vi "Error Dialog.vi"(6 "Modal (T)":bool=TRUE, 8 "error in (no error)":errorcluster, 10 "Dialog Type":T1) -> (0 "error out":errorcluster)   [LabVIEW 2017, in "Error Dialog w Copy to Clipboard.lvlib"]
doc: "Displays error message to the user.\n\nCopyright (c) 2022, Neosoft Technologies Inc\nAll rights reserved."
uses:
  Error Dialog w Copy to Clipboard.lvlib
  Dialog Type.ctl
  <vilib>/Utility/error.llb/DialogType.ctl
  <vilib>/Platform/browser.llb/Open URL in Default Browser (string).vi
panel:
  out "String":string
  in  "Stop":bool
  in  "Continue":bool
  out "Error Code":string
  in  "Show details":bool
  in  "Screenshot":bool
  in  "URL":bool
  in  "Copy":bool
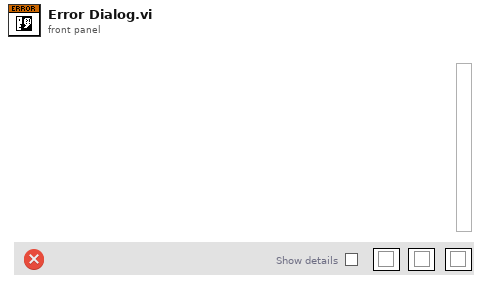
[diagram p1: front panel]
types:
  T1 = typedef "Error Dialog w Copy to Clipboard.lvlib/Dialog Type.ctl" = enum16{"OK message", "Continue or Stop message"}
  T2 = enum32{"Invalid", "Default", "Floating", "Floating/Auto-Hide", "Modal"}
  T3 = enum32{"Invalid", "Standard", "Closed", "Hidden", "Minimized", "Maximized"}
  T4 = cluster{"call chain":string[], "error":errorcluster, "show details":bool, "message":string, "stop":bool}
  T5 = typedef "imagedata.ctl" = cluster{"image type":i32, "image depth":i32, "image":u8[], "mask":u8[], "colors":u32[], "Rectangle":cluster{"left":i16, "top":i16, "right":i16, "bottom":i16}}
  T6 = typedef "DialogType.ctl" = u16
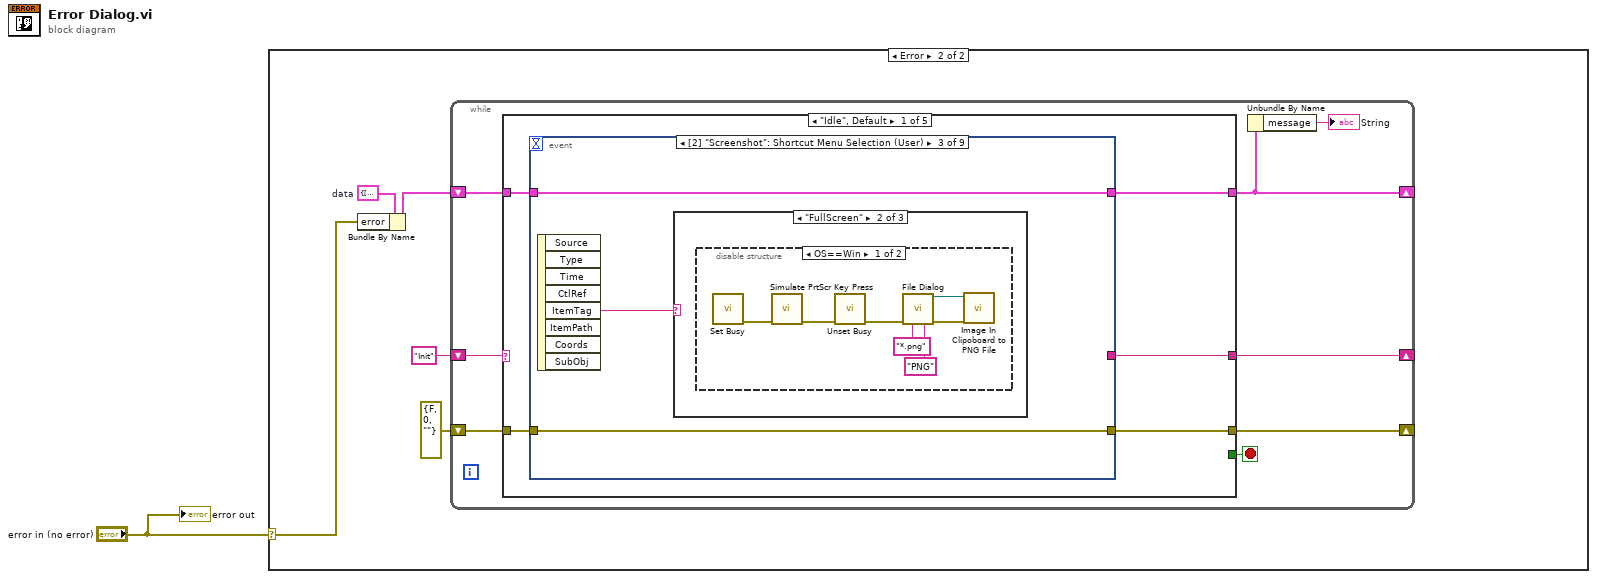
[diagram p0: block diagram]
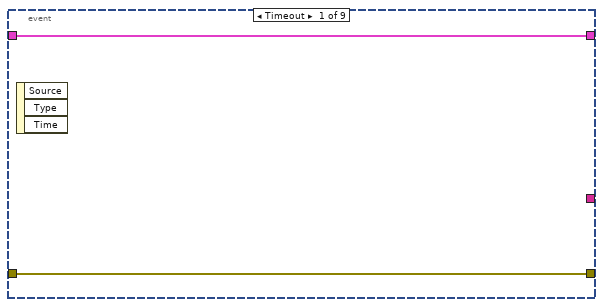
[diagram p3: hidden frame]
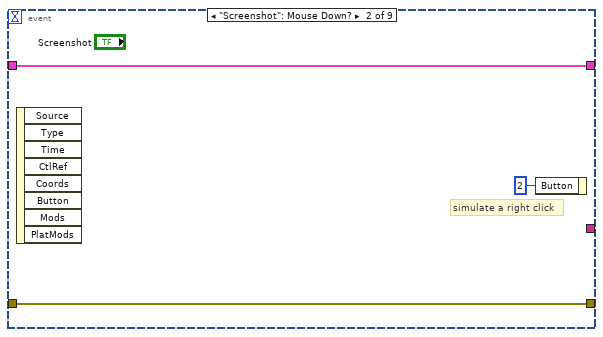
[diagram p4: hidden frame]
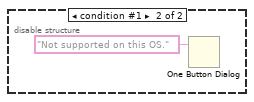
[diagram p6: hidden frame]
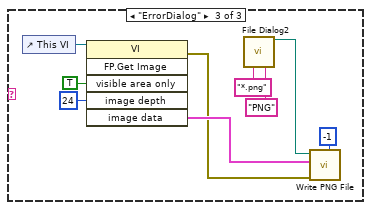
[diagram p7: hidden frame]
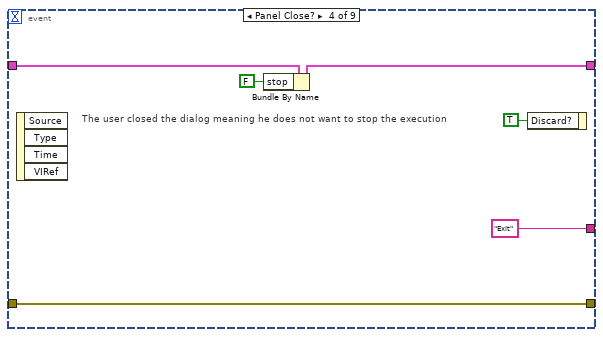
[diagram p8: hidden frame]
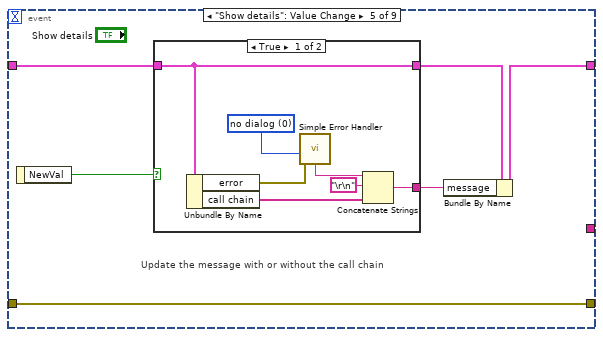
[diagram p9: hidden frame]
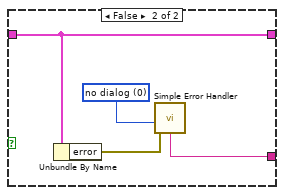
[diagram p10: hidden frame]
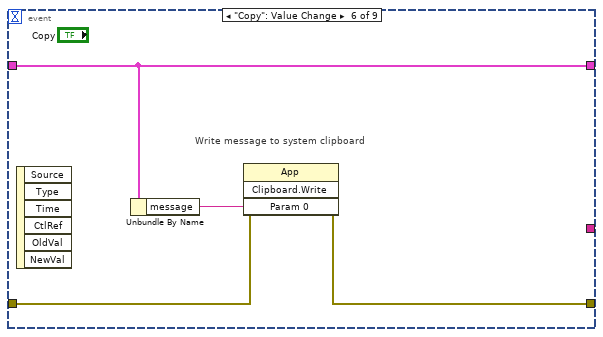
[diagram p11: hidden frame]
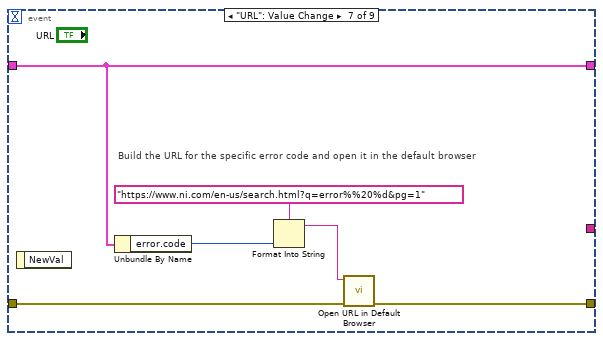
[diagram p12: hidden frame]
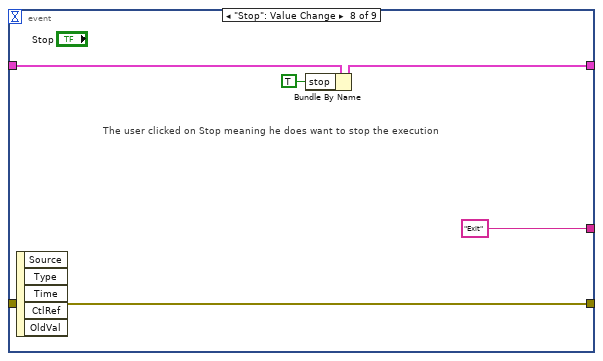
[diagram p13: hidden frame]
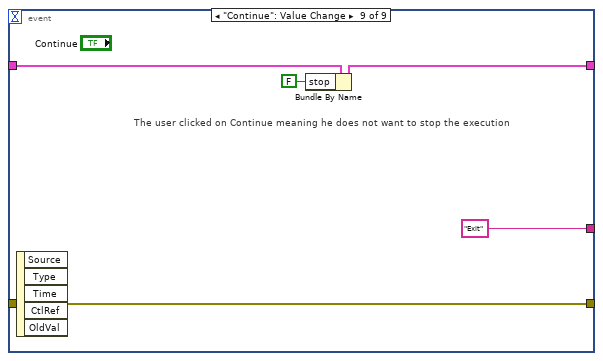
[diagram p14: hidden frame]
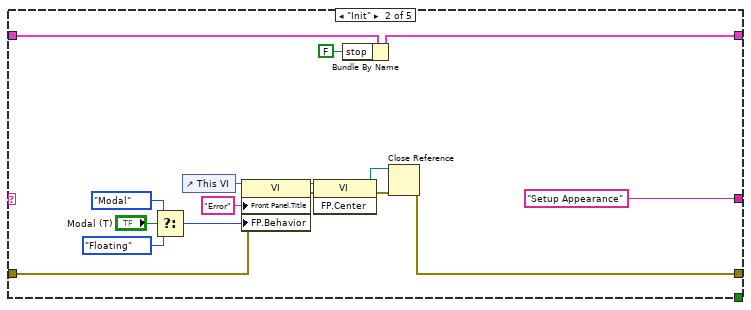
[diagram p15: hidden frame]
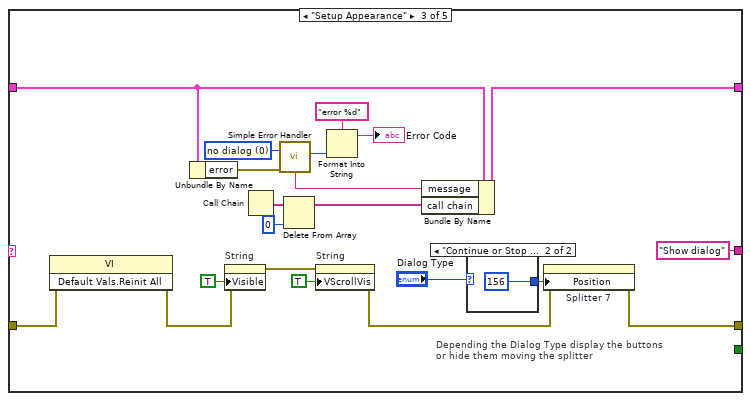
[diagram p16: hidden frame]
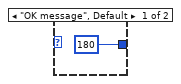
[diagram p17: hidden frame]
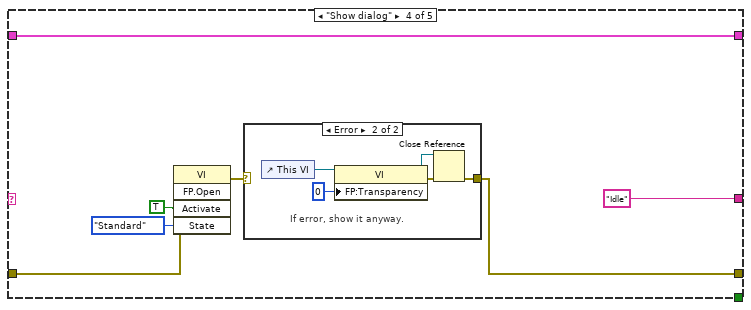
[diagram p18: hidden frame]
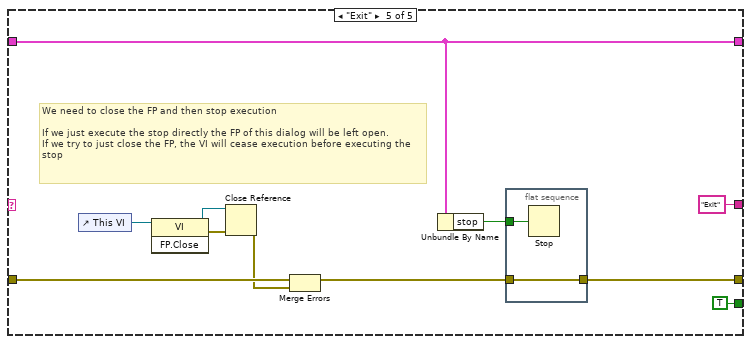
[diagram p20: hidden frame]
diagram:
  n1 = case shown="Error" "error in (no error)" {
    selector: "error in (no error)" -> [_ w3]
    frame No Error {
    }
    frame Error {
      w5 = T4 {"call chain"=[], "error"={"status"=FALSE, "code"=0, "source"=""}, "show details"=FALSE, "message"="", "stop"=FALSE}  # data
      n2 = Bundle By Name(cluster=w5, "error"=w3) -> (w4:T4)
      n3 = while {
        shift-right: [w12] -> _
        shift-left: "Init" ("format string") -> [w13]
        shift-right: [w11] -> _
        shift-left: errorcluster {"status"=FALSE, "code"=0, "source"=""} ("error out") -> [w10]
        shift-right: [w8] -> _
        shift-left: w4 -> [w9]
        stop <- w14 stop-if-true
        n4 = case shown="\"Idle\", Default" w13 {
          tunnel: [_ _ _ _ TRUE ("Discard?")] -> w14
          tunnel: [w15 "Setup Appearance" "Show dialog" "Idle" "Exit" ("format string")] -> w12
          tunnel: [w18 w96 w104 w127 w142] -> w11
          tunnel: w10 -> [w19 w95 w109 w128 w149]
          tunnel: [w16 w89 w115 w133 w144] -> w8
          tunnel: w9 -> [w17 w94 w123 w133 w144]
          frame "Idle", Default {
            n5 = event shown="[2] \"Screenshot\": Shortcut Menu Selection (User)" {
              selector: _ -> [_ _ _ _ _ _ _ _ _]
              dyn-events: _ -> [_ _ _ _ _ _ _ _ _]
              timeout: _ -> [_ _ _ _ _ _ _ _ _]
              tunnel: w19 -> [w21 w22 w27 w50 w56 w69 w73 w82 w87]
              tunnel: [w21 w22 w27 w50 w56 w68 w72 w82 w87] -> w18
              tunnel: w17 -> [w20 w24 w26 w49 w54 w71 w77 w81 w86]
              tunnel: [w20 w24 w26 w46 w52 w71 w77 w80 w85] -> w16
              tunnel: [_ _ _ "Exit" ("format string") _ _ _ "Exit" ("format string") "Exit" ("format string")] -> w15
              event Timeout {
                n6 = event-data() -> ()  [unwired: 1 in, 3 out]
              }
              event "Screenshot": Mouse Down? {
                # "simulate a right click"
                n7 = event-data() -> ()  [unwired: 1 in, 8 out]
                n8 = event-data("Button"=u16 2) -> ()  [unwired: 1 in, 1 out]
              }
              event "Screenshot": Shortcut Menu Selection (User) {
                n9 = event-data() -> ("ItemTag"=w25:string)  [unwired: 1 in, 7 out]
                n10 = case shown="\"FullScreen\"" w25 {
                  frame "False", Default {
                  }
                  frame "FullScreen" {
                    n11 = disable-structure shown="OS==Win" {
                      frame condition #0 (active) {
                        n12 = call <vilib>:"Set Busy.vi"() -> ("error out"=w30:errorcluster)  [unwired: 10 in, 1 out]
                        n13 = call "Simulate PrtScr Key Press.vi"("error in (no error)"=w30) -> ("error out"=w29:errorcluster)  [unwired: 10 in]
                        n14 = call <vilib>:"Unset Busy.vi"("error in (no error)"=w29) -> ("error out"=w28:errorcluster)  [unwired: 10 in]
                        n15 = call "File Dialog"("error in"=w28, "pattern (all files)"="*.png", "pattern label"="PNG") -> ("selected path"=w34:path, "error out"=w31:errorcluster)  [unwired: 9 in, 2 out]
                        n16 = call "Image In Clipoboard to PNG File.vi"("error in (no error)"=w31, "Image Path"=w34) -> ()  [unwired: 9 in, 1 out]
                      }
                      frame condition #1 {
                        n17 = One Button Dialog(message="Not supported on this OS.") -> ()  [unwired: 1 in, 1 out]
                      }
                    }
                  }
                  frame "ErrorDialog" {
                    n18 = control-ref of="This VI"() -> (w44:refnum<vi>)
                    n19 = invoke class="VI" method="FP.Get Image"(reference=w44, "visible area only"=TRUE ("Visible Area Only"), "image depth"=24 ("Image Depth")) -> (error out=w42:errorcluster, "image data"=w43:T5)  [unwired: 3 in, 4 out]
                    n20 = call "File Dialog2"("pattern (all files)"="*.png", "pattern label"="PNG") -> ("selected path"=w36:path)  [unwired: 10 in, 3 out]
                    n21 = call <vilib>:"Write PNG File.vi"("compression (default)"=-1, "error in (no error)"=w42, "image data"=w43, "path to PNG file"=w36) -> ()  [unwired: 6 in, 2 out]
                  }
                }
              }
              event Panel Close? {
                # "The user closed the dialog meaning he does not want to stop the execution"
                n22 = event-data() -> ()  [unwired: 1 in, 4 out]
                n23 = Bundle By Name(cluster=w49, "stop"=FALSE) -> (w46:T4)
                n24 = event-data("Discard?"=TRUE) -> ()  [unwired: 1 in, 1 out]
              }
              event "Show details": Value Change {
                # "Update the message with or without the call chain"
                n25 = event-data() -> ("NewVal"=w55:bool)  [unwired: 1 in]
                n26 = case shown="True" w55 {
                  tunnel: w54 -> [w61 w65]
                  tunnel: [w61 w65] -> w53
                  tunnel: [w57 w64] -> w51
                  frame True {
                    w60 = "\r\n"
                    w63 = T6 0 items=["no dialog", "OK message", "continue or stop message", "OK message + warnings", "continue/stop + warnings"] ("type of dialog (OK msg:1)")
                    n27 = Unbundle By Name(w61) -> ("error"=w62:errorcluster, "call chain"=w58:string[])
                    n28 = call <vilib>:"Simple Error Handler.vi"("type of dialog (OK msg:1)"=w63, "error in (no error)"=w62) -> ("message"=w59:string)  [unwired: 3 in, 4 out]
                    n29 = Concatenate Strings(w59, w60, w60, w58) -> (w57:string)
                  }
                  frame False {
                    w67 = T6 0 items=["no dialog", "OK message", "continue or stop message", "OK message + warnings", "continue/stop + warnings"] ("type of dialog (OK msg:1)")
                    n30 = Unbundle By Name(w65) -> ("error"=w66:errorcluster)
                    n31 = call <vilib>:"Simple Error Handler.vi"("type of dialog (OK msg:1)"=w67, "error in (no error)"=w66) -> ("message"=w64:string)  [unwired: 3 in, 4 out]
                  }
                }
                n32 = Bundle By Name(cluster=w53, "message"=w51) -> (w52:T4)
              }
              event "Copy": Value Change {
                # "Write message to system clipboard"
                n33 = event-data() -> ()  [unwired: 1 in, 6 out]
                n34 = Unbundle By Name(w71) -> ("message"=w70:string)
                n35 = invoke class="App" method="Clipboard.Write"(error in=w69, "Param 0"=w70) -> (error out=w68:errorcluster)  [unwired: 2 in, 3 out]
              }
              event "URL": Value Change {
                # "Build the URL for the specific error code and open it in the default browser"
                n36 = event-data() -> ()  [unwired: 1 in, 1 out]
                n37 = Unbundle By Name(w77) -> ("error.code"=w75:i32)
                n38 = Format Into String(format string="https://www.ni.com/en-us/search.html?q=error%%20%d&pg=1", w75) -> (resulting string=w74:string)  [unwired: 2 in, 1 out]
                n39 = call-poly <vilib>:"Open URL in Default Browser.vi"("error in (no error)"=w73, "URL"=w74) -> ("error out"=w72:errorcluster)  [unwired: 4 in, 1 out]
              }
              event "Stop": Value Change {
                # "The user clicked on Stop meaning he does want to stop the execution"
                n40 = event-data() -> ()  [unwired: 1 in, 5 out]
                n41 = Bundle By Name(cluster=w81, "stop"=TRUE) -> (w80:T4)
              }
              event "Continue": Value Change {
                # "The user clicked on Continue meaning he does not want to stop the execution"
                n42 = event-data() -> ()  [unwired: 1 in, 5 out]
                n43 = Bundle By Name(cluster=w86, "stop"=FALSE) -> (w85:T4)
              }
            }
          }
          frame "Init" {
            n44 = Select(t=T2."Modal" ("Front Panel Window:Behavior"), s="Modal (T)", f=T2."Floating") -> (s? t:f=w90:T2)
            n45 = control-ref of="This VI"() -> (w101:refnum<vi>)
            n46 = property class="VI"(reference=w101, error in=w95, "Front Panel.Title"="Error" ("Front Panel Window:Title"), "FP.Behavior"=w90) -> (reference out=w102:refnum<vi>, error out=w103:errorcluster)
            n47 = invoke class="VI" method="FP.Center"(reference=w102, error in=w103) -> (reference out=w99:refnum<vi>, error out=w98:errorcluster)  [unwired: 1 in, 1 out]
            n48 = Bundle By Name(cluster=w94, "stop"=FALSE) -> (w89:T4)
            n49 = Close Reference(reference=w99, error in (no error)=w98) -> (error out=w96:errorcluster)
          }
          frame "Setup Appearance" {
            w121 = T6 0 items=["no dialog", "OK message", "continue or stop message", "OK message + warnings", "continue/stop + warnings"] ("type of dialog (OK msg:1)")
            # "Depending the Dialog Type display the buttons or hide them moving the splitter"
            n50 = invoke class="VI" method="Default Vals.Reinit All"(error in=w109) -> (error out=w108:errorcluster)  [unwired: 2 in, 2 out]
            n51 = Unbundle By Name(w123) -> ("error"=w122:errorcluster)
            n52 = property on="String" class="Str"(error in=w108, "Visible"=TRUE) -> (error out=w117:errorcluster)  [unwired: 1 in, 1 out]
            n53 = Call Chain() -> (call chain=w112:string[])
            n54 = call <vilib>:"Simple Error Handler.vi"("type of dialog (OK msg:1)"=w121, "error in (no error)"=w122) -> ("code out"=w120:i32, "message"=w114:string)  [unwired: 3 in, 3 out]
            n55 = Delete From Array(array=w112, index=0) -> (array with subset deleted=w111:string[])  [unwired: 1 in, 1 out]
            n56 = property on="String" class="Str"(error in=w117, "VScrollVis"=TRUE ("Vertical Scrollbar Visible")) -> (error out=w105:errorcluster)  [unwired: 1 in, 1 out]
            n57 = Format Into String(format string="error %d", w120) -> (resulting string=→"Error Code":string)  [unwired: 2 in, 1 out]
            n58 = Bundle By Name(cluster=w123, "message"=w114, "call chain"=w111) -> (w115:T4)
            n59 = case shown="\"Continue or Stop message\"" "Dialog Type" {
              tunnel: [180 156] -> w106
              frame "OK message", Default {
              }
              frame "Continue or Stop message" {
              }
            }
            n60 = property on="Splitter 7" class="Splitter"(error in=w105, "Position"=w106) -> (error out=w104:errorcluster)  [unwired: 1 in, 1 out]
          }
          frame "Show dialog" {
            n61 = invoke class="VI" method="FP.Open"(error in=w128, "Activate"=TRUE ("Front Panel Window:Open"), "State"=T3."Standard") -> (error out=w131:errorcluster)  [unwired: 2 in, 4 out]
            n62 = case shown="Error" w131 {
              selector: w131 -> [w134 _]
              tunnel: [w134 w135] -> w127
              frame No Error {
              }
              frame Error {
                # "If error, show it anyway."
                n63 = control-ref of="This VI"() -> (w137:refnum<vi>)
                n64 = property class="VI"(reference=w137, "FP:Transparency"=u8 0 ("Front Panel Window:Transparency")) -> (reference out=w138:refnum<vi>, error out=w139:errorcluster)  [unwired: 1 in]
                n65 = Close Reference(reference=w138, error in (no error)=w139) -> (error out=w135:errorcluster)
              }
            }
          }
          frame "Exit" {
            # "We need to close the FP and then stop execution\n\nIf we just execute the stop directly the FP of this dialog will be left open.\nIf we try to just close the FP, the VI will cease execution before executing the stop"
            n66 = control-ref of="This VI"() -> (w148:refnum<vi>)
            n67 = invoke class="VI" method="FP.Close"(reference=w148) -> (reference out=w146:refnum<vi>, error out=w147:errorcluster)  [unwired: 2 in, 1 out]
            n68 = Close Reference(reference=w146, error in (no error)=w147) -> (error out=w145:errorcluster)
            n69 = Merge Errors(w149, w145) -> (w143:errorcluster)
            n70 = Unbundle By Name(w144) -> ("stop"=w141:bool)
            n71 = flat-sequence {
              tunnel: w143 -> [w152]
              tunnel: [w152] -> w142
              tunnel: w141 -> [w151]
              frame #0 {
                n72 = Stop(stop? (T)=w151) -> ()
              }
            }
          }
        }
        n73 = Unbundle By Name(w8) -> ("message"=→"String":string)
      }
    }
  }
  "error out" <- "error in (no error)"
